vi "WriteData.vi"(8 "Error In":errorcluster, 10 "Data":string, 11 "reference in":refnum<class "EncryptedFileDataSource.lvclass">) -> (0 "Error Out":errorcluster, 3 "reference in":refnum<class "EncryptedFileDataSource.lvclass">)   [LabVIEW 2020, in "EncryptedFileDataSource.lvclass"]
uses:
  EncryptedFileDataSource.lvclass
  FileDataSource_class/FileDataSource.lvclass
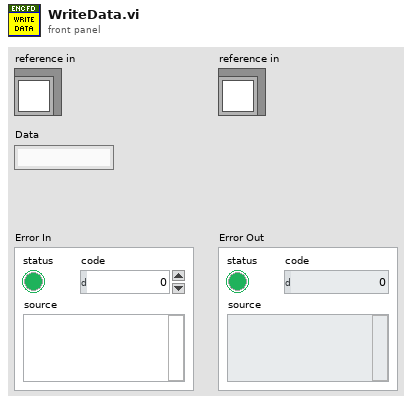
[diagram p1: front panel]
types:
  T1 = typedef "EncryptedFileDataSource.lvclass/ObjectAttributes.ctl" = cluster{"EncryptionType":T2}
  T2 = typedef "EncryptedFileDataSource.lvclass/EncryptionType.ctl" = enum16{"Type 1", "Type 2"}
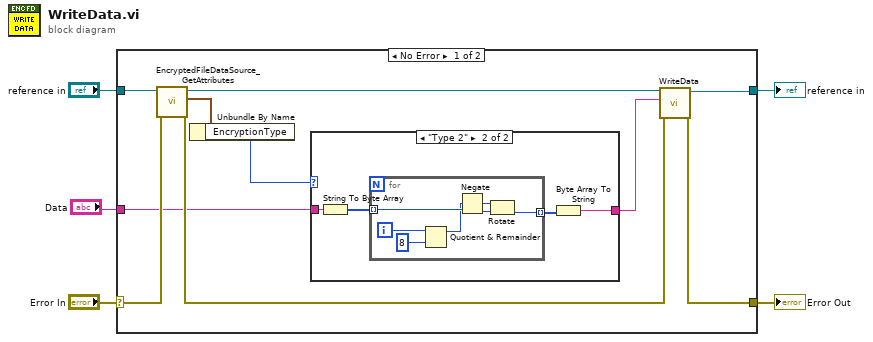
[diagram p0: block diagram]
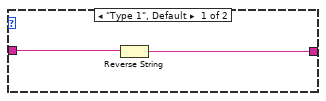
[diagram p2: hidden frame]
diagram:
  n1 = case shown="No Error" "Error In" {
    selector: "Error In" -> [w15 w29]
    tunnel: [w9 w29] -> w4
    tunnel: [w11 w28] -> w2
    tunnel: "reference in" -> [w13 w28]
    tunnel: "Data" -> [w7 _]
    frame No Error {
      n2 = call "EncryptedFileDataSource_GetAttributes.vi"("error in (no error)"=w15, "reference in"=w13) -> ("error out"=w10:errorcluster, "Data"=w14:T1, "reference out"=w12:refnum<class "EncryptedFileDataSource.lvclass">)  [unwired: 6 in, 1 out]
      n3 = Unbundle By Name(w14) -> ("EncryptionType"=w8:T2)
      n4 = case shown="\"Type 2\"" w8 {
        tunnel: w7 -> [w17 w19]
        tunnel: [w16 w18] -> w6
        frame "Type 1", Default {
          n5 = Reverse String(1:w17) -> (0:w16:string)
        }
        frame "Type 2" {
          n6 = String To Byte Array(string=w19) -> (unsigned byte array=w20:u8[])
          n7 = for {
            tunnel: w20 -> [w25] mode=indexing
            tunnel: [w24] -> w21 mode=indexing
            i -> [w27]
            n8 = Quotient & Remainder(x=w27, y=8) -> (x-y*floor(x/y)=w23:i32)  [unwired: 1 out]
            n9 = Negate(x=w23) -> (-x=w22:i32)
            n10 = Rotate(1:w25, 2:w22) -> (0:w24:u8)
          }
          n11 = Byte Array To String(unsigned byte array=w21) -> (string=w18:string)
        }
      }
      n12 = call-parent "WriteData.vi"("Error In"=w10, "Data"=w6, "reference in"=w12) -> ("Error Out"=w9:errorcluster, "reference out"=w11:refnum<class "EncryptedFileDataSource.lvclass">)  [unwired: 7 in]
    }
    frame Error {
    }
  }
  "Error Out" <- w4
  "reference in" <- w2
